vi "Set Last Temperatures.vi"(6 "Read Channel Ident":string, 8 "error in":errorcluster, 9 "Temperatures":dbl[][](array[numeric]), 10 "Channel Idents":string[](array[string]), 11 "Thermometer DAQmx RTD Cont CFG in":refnum<class "Thermometer DAQmx RTD Cont CFG.lvclass">) -> (0 "error out":errorcluster, 1 "Temperature":dbl, 3 "Thermometer DAQmx RTD Cont CFG out":refnum<class "Thermometer DAQmx RTD Cont CFG.lvclass">)   [LabVIEW 2024, in "Thermometer DAQmx RTD Cont CFG.lvclass"]
uses:
  Thermometer DAQmx RTD Cont CFG.lvclass
  Thermometer DAQmx RTD Cont CFG.lvclass/Thermometer DAQmx RTD Cont CFG.ctl
  <vilib>/Analysis/baseanly.llb/Mean (DBL).vi
  <vilib>/Analysis/NI_AALBase.lvlib
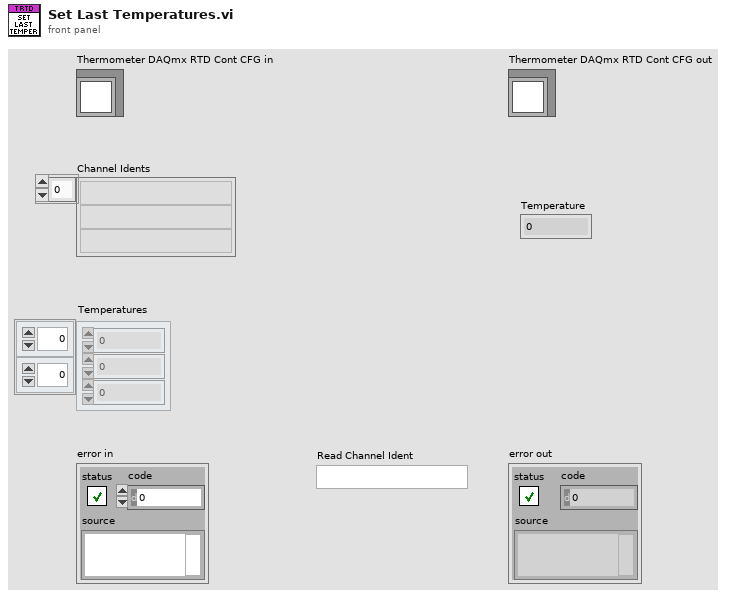
[diagram p1: front panel]
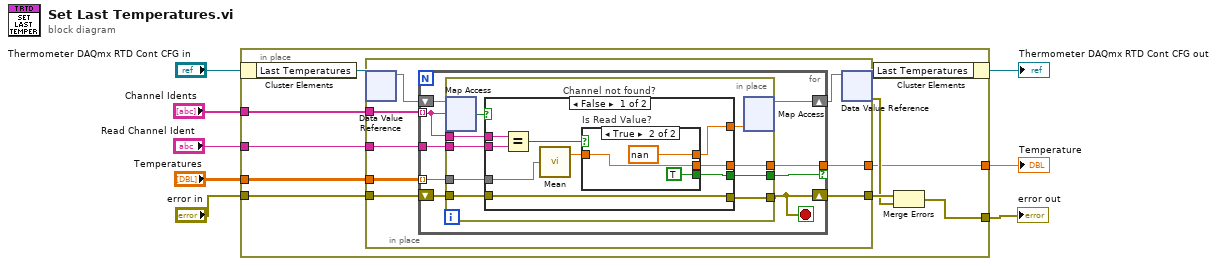
[diagram p0: block diagram]
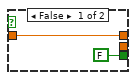
[diagram p2: hidden frame]
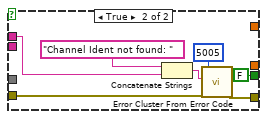
[diagram p3: hidden frame]
diagram:
  n1 = in-place {
    in-place-border: "Temperatures" -> [w17]
    in-place-border: "error in" -> [w16]
    in-place-border: [w13] -> w7
    in-place-border: "Channel Idents" -> [w11]
    in-place-border: "Read Channel Ident" -> [w10]
    in-place-border: [w9] -> w1
    n2 = in-place-cluster #1("Thermometer DAQmx RTD Cont CFG in") -> ("Last Temperatures"=w18:refnum<data-value>)
    n3 = in-place {
      in-place-border: w17 -> [w25]
      in-place-border: w16 -> [w26]
      in-place-border: [w24] -> w15
      in-place-border: w11 -> [w22]
      in-place-border: w10 -> [w20]
      in-place-border: [w19] -> w9
      n4 = in-place-dvr #2(w18) -> (w23:map{string, dbl})  [unwired: 1 out]
      n5 = for {
        tunnel: w25 -> [w34] mode=indexing
        shift-right: [w27] -> w24
        shift-left: w26 -> [w35]
        tunnel: w22 -> [w32] mode=indexing
        shift-right: [w31] -> w21
        shift-left: w23 -> [w33]
        tunnel: w20 -> [w30]
        tunnel: [w29] -> w19 if=w28
        stop <- w27 stop-if-true
        n6 = in-place {
          in-place-border: w35 -> [w44]
          in-place-border: w34 -> [w43]
          in-place-border: [w42] -> w27
          in-place-border: w32 -> [w40]
          in-place-border: w30 -> [w39]
          in-place-border: [w37] -> w29
          in-place-border: [w36] -> w28
          n7 = in-place-map #3(w33, w32) -> (w41:bool)  [unwired: 1 in, 1 out]
          n8 = case "Channel not found?" shown="False" w41 {
            tunnel: w44 -> [w53 w65]
            tunnel: w43 -> [w47 _]
            tunnel: [w53 w61] -> w42
            tunnel: w40 -> [w51 w60]
            tunnel: w39 -> [w52 _]
            tunnel: [w46 _] -> w38
            tunnel: [w49 _] -> w37
            tunnel: [w45 FALSE] -> w36
            frame False {
              n9 = Equal?(x=w51, y=w52) -> (x = y?=w50:bool)
              n10 = call-poly <vilib>:"Mean.vi"("X"=w47) -> ("mean"=w48:dbl)  [unwired: 1 out]
              n11 = case "Is Read Value?" shown="True" w50 {
                tunnel: [w55 nan] -> w46
                tunnel: [_ w57] -> w49
                tunnel: w48 -> [w55 w57]
                tunnel: [FALSE TRUE] -> w45
                frame False {
                }
                frame True {
                }
              }
            }
            frame True {
              n12 = Concatenate Strings("Channel Ident not found: " ("error message (\"\")"), w60) -> (w63:string)
              n13 = call <vilib>:"Error Cluster From Error Code.vi"("error in (no error)"=w65, "error message (\"\")"=w63, "error code (0)"=5005) -> ("error out"=w61:errorcluster)  [unwired: 6 in]
            }
          }
          n14 = in-place-map #3(w38) -> (w31:map{string, dbl})  [unwired: 1 in, 2 out]
        }
      }
      n15 = in-place-dvr #2(w21) -> (w14:refnum<data-value>, w12:errorcluster)
    }
    n16 = in-place-cluster #1("Last Temperatures"=w14) -> (→"Thermometer DAQmx RTD Cont CFG out":refnum<class "Thermometer DAQmx RTD Cont CFG.lvclass">)
    n17 = Merge Errors(w15, w12) -> (w13:errorcluster)
  }
  "error out" <- w7
  "Temperature" <- w1
